vi "Configure Limit Test Result Pattern.vi"(0 "VISA resource name":refnum<visa-resource-name>, 1 "Limit Test Upper Exceeding Pattern (0)":i32, 2 "Limit Test Pass Pattern (0)":i32, 5 "Channel (1: Channel 1)":i32(ring)=1 items=["Channel 1"=1, "Channel 2"=2], 9 "Limit Test Number (1)":i32=1, 11 "error in (no error)":errorcluster, 12 "Limit Test Lower Exceeding Pattern (0)":i32, 13 "Limit Test Failure Pattern (0)":i32) -> (4 "VISA resource name out":refnum<visa-resource-name>, 15 "error out":errorcluster)   [LabVIEW 2012, in "Keysight B2980 Series.lvlib"]
doc: "Configures bit patterns used to indicate different limit test results."
uses:
  Keysight B2980 Series.lvlib
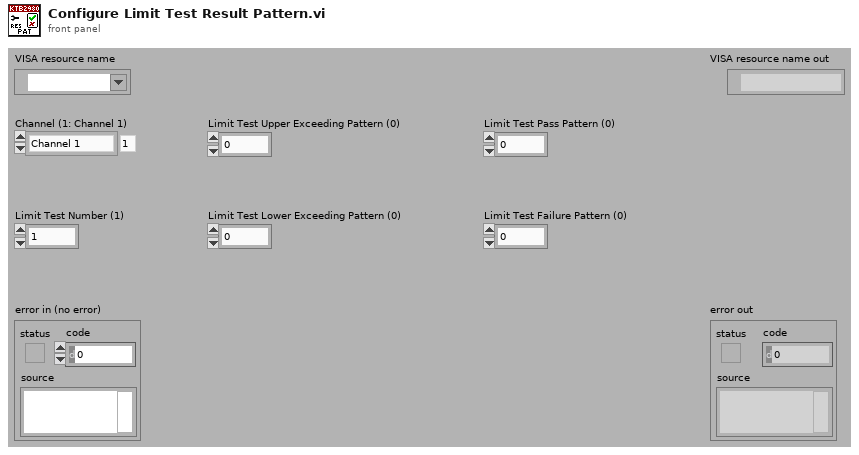
[diagram p1: front panel]
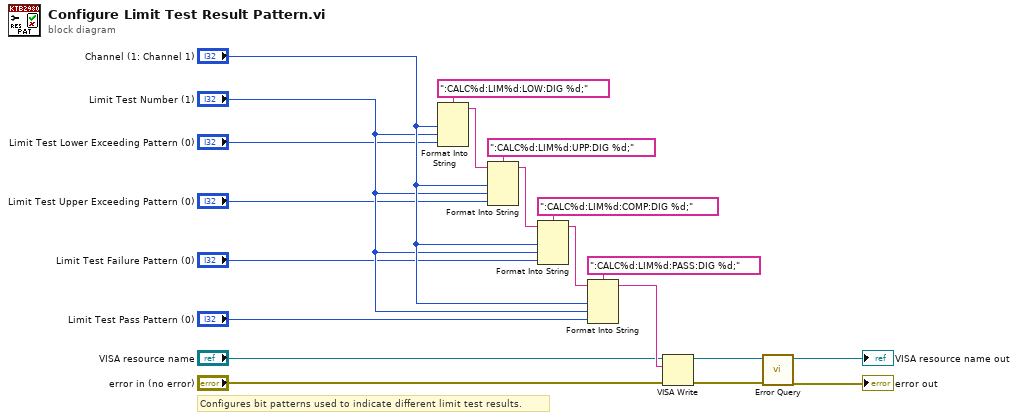
[diagram p0: block diagram]
diagram:
  # "Configures bit patterns used to indicate different limit test results."
  n1 = Format Into String(format string=":CALC%d:LIM%d:LOW:DIG %d;", "Channel (1: Channel 1)", "Limit Test Number (1)", "Limit Test Lower Exceeding Pattern (0)") -> (resulting string=w16:string)  [unwired: 2 in, 1 out]
  n2 = Format Into String(format string=":CALC%d:LIM%d:UPP:DIG %d;", initial string=w16, "Channel (1: Channel 1)", "Limit Test Number (1)", "Limit Test Upper Exceeding Pattern (0)") -> (resulting string=w13:string)  [unwired: 1 in, 1 out]
  n3 = Format Into String(format string=":CALC%d:LIM%d:COMP:DIG %d;", initial string=w13, "Channel (1: Channel 1)", "Limit Test Number (1)", "Limit Test Failure Pattern (0)") -> (resulting string=w10:string)  [unwired: 1 in, 1 out]
  n4 = Format Into String(format string=":CALC%d:LIM%d:PASS:DIG %d;", initial string=w10, "Channel (1: Channel 1)", "Limit Test Number (1)", "Limit Test Pass Pattern (0)") -> (resulting string=w7:string)  [unwired: 1 in, 1 out]
  n5 = VISA Write(VISA resource name="VISA resource name", write buffer=w7, error in (no error)="error in (no error)") -> (VISA resource name out=w4:refnum<visa-resource-name>, error out=w3:errorcluster)  [unwired: 1 out]
  n6 = call "Error Query.vi"("error in (no error)"=w3, "VISA resource name"=w4) -> ("error out"=→"error out":errorcluster, "VISA resource name out"=→"VISA resource name out":refnum<visa-resource-name>)  [unwired: 8 out]
